vi "Close.vi"(8 "error in":errorcluster, 11 "Red-y Read Write CFG in":refnum<class "Red-y Pressure Control CFG.lvclass">) -> (0 "error out":errorcluster, 3 "Red-y Read Write CFG out":refnum<class "Red-y Pressure Control CFG.lvclass">)   [LabVIEW 2024, in "Red-y Pressure Control CFG.lvclass"]
uses:
  Red-y Pressure Control CFG.lvclass
  Red-y Pressure Control CFG.lvclass/Red-y Pressure Control CFG.ctl
  Voegtlin_NI_SMART_Modbus_Drivers/Voegtlin_NI_SMART_Modbus_Drivers.lvlib
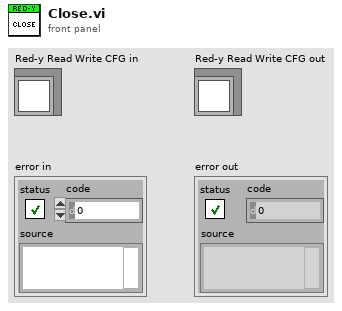
[diagram p1: front panel]
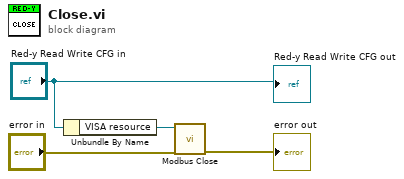
[diagram p0: block diagram]
diagram:
  n1 = Unbundle By Name("Red-y Read Write CFG in") -> ("VISA resource"=w1:refnum<visa-resource-name>)
  n2 = call "Modbus Close.vi"("error in (no error)"="error in", "VISA resource in"=w1) -> ("error out"=→"error out":errorcluster)  [unwired: 9 in]
  "Red-y Read Write CFG out" <- "Red-y Read Write CFG in"
